vi "Run_Core.vi"(0 "For Loop in":refnum<class "Structure If Else.lvclass">, 11 "error in (no error)":errorcluster) -> (4 "For Loop out":refnum<class "Structure If Else.lvclass">, 6 "Return":variant, 15 "error out":errorcluster)   [LabVIEW 2019, in "Structure If Else.lvclass"]
uses:
  Structure If Else.lvclass
  Structure If Else.lvclass/Structure If Else.ctl
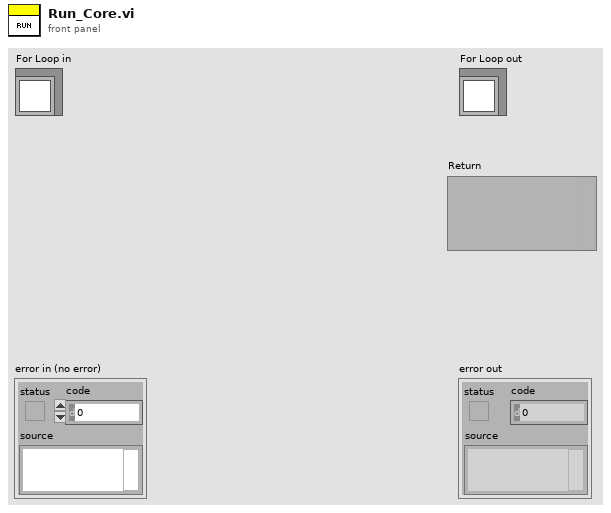
[diagram p1: front panel]
types:
  T1 = typedef "Structure If Else.lvclass/function list.ctl" = enum16{"if", "elif", "else"}
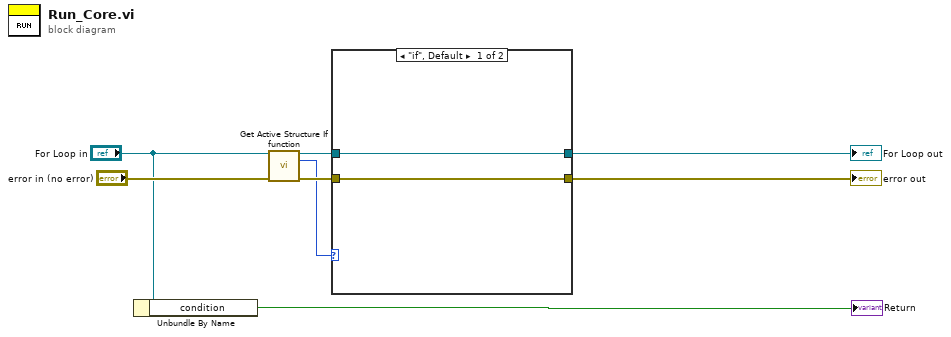
[diagram p0: block diagram]
diagram:
  n1 = Unbundle By Name("For Loop in") -> ("condition"=→"Return":bool)
  n2 = call "Get Active Structure If function.vi"("Structure If Else in"="For Loop in", "error in (no error)"="error in (no error)") -> ("Structure If Else out"=w2:refnum<class "Structure If Else.lvclass">, "function list"=w1:T1, "error out"=w4:errorcluster)  [unwired: 11 in]
  n3 = case shown="\"if\", Default" w1 {
    tunnel: w2 -> [w10 w12]
    tunnel: [w10 w12] -> w8
    tunnel: w4 -> [w9 w11]
    tunnel: [w9 w11] -> w7
    frame "if", Default {
    }
    frame "elif" {
    }
  }
  "error out" <- w7
  "For Loop out" <- w8
